vi "UTILITY 1D String to 1D Integer.vi"(11 "1D String":string[](array[string])) -> (3 "1D Integer":i32[](array[numeric]))   [LabVIEW 2016]
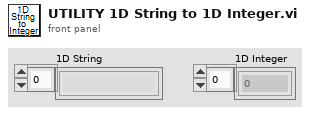
[diagram p1: front panel]
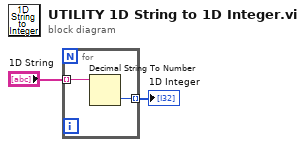
[diagram p0: block diagram]
diagram:
  n1 = for {
    tunnel: "1D String" -> [w4] mode=indexing
    tunnel: [w3] -> w2 mode=indexing
    n2 = Decimal String To Number(string=w4) -> (number=w3:i32)  [unwired: 2 in, 1 out]
  }
  "1D Integer" <- w2
